vi "Open Document.vi"(7 "xwpfDocument Type":refnum<class "xwpfDocument.lvclass">, 8 "error in (no error)":errorcluster, 11 "Document Path":path) -> (0 "error out":errorcluster, 3 "xwpfDocument out":refnum<class "xwpfDocument.lvclass">)   [LabVIEW 2017, in "Word_Specific.lvlib" / "xwpfDocument.lvclass"]
uses:
  xwpfDocument.lvclass
  C:/Users/Neo/Desktop/Dev_Tools_BR/LabVIEW_NPOI/src/lib/NPOI 2.1.1/NPOI.OOXML.dll
  lib/NPOI 2.1.1/NPOI.OOXML.dll
  xwpfDocument.lvclass/xwpfDocument.ctl
  Support/File Stream/File Stream.lvlib
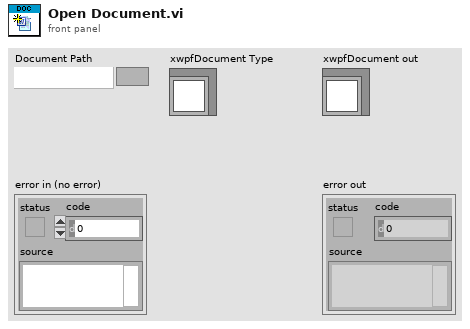
[diagram p1: front panel]
types:
  T1 = enum16{"Title", "Heading 1", "Heading 2", "Heading 3", "Normal", "Figure", "Page Break"}
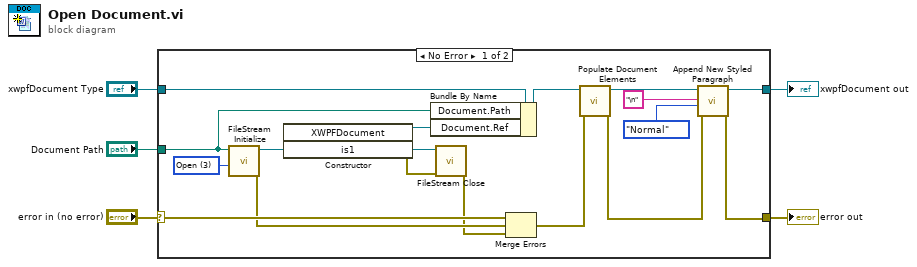
[diagram p0: block diagram]
diagram:
  n1 = case shown="No Error" "error in (no error)" {
    selector: "error in (no error)" -> [w21 w24]
    tunnel: [w8 w24] -> w4
    tunnel: [w10 w23] -> w2
    tunnel: "xwpfDocument Type" -> [w22 w23]
    tunnel: "Document Path" -> [w11 _]
    frame No Error {
      w20 = 3 items=["CreateNew"=1, "Create"=2, "Open"=3, "OpenOrCreate"=4, "Truncate"=5, "Append"=6] ("mode")
      n2 = call "FileStream Initialize.vi"("mode"=w20, "path"=w11) -> ("error out"=w16:errorcluster, "new reference"=w18:refnum<k24>)  [unwired: 8 in]
      n3 = constructor class="XWPFDocument"("is1"=w18) -> (reference out=w19:refnum<k24>, error out=w17:errorcluster)  [unwired: 3 in, 2 out]
      n4 = Bundle By Name(cluster=w22, "Document.Path"=w11, "Document.Ref"=w19) -> (w14:refnum<class "xwpfDocument.lvclass">)
      n5 = call "FileStream Close.vi"("error in (no error)"=w17, "reference"=w18) -> ("error out"=w15:errorcluster)  [unwired: 9 in]
      n6 = Merge Errors(w21, w16, w15) -> (w12:errorcluster)
      n7 = call "Populate Document Elements.vi"("error in (no error)"=w12, "xwpfDocument in"=w14) -> ("error out"=w9:errorcluster, "xwpfDocument out"=w13:refnum<class "xwpfDocument.lvclass">)  [unwired: 8 in]
      n8 = call "Append New Styled Paragraph.vi"("error in (no error)"=w9, "Type"=T1."Normal", "Paragraph.Text"="\n", "xwpfDocument in"=w13) -> ("error out"=w8:errorcluster, "xwpfDocument out"=w10:refnum<class "xwpfDocument.lvclass">)  [unwired: 6 in]
    }
    frame Error {
    }
  }
  "error out" <- w4
  "xwpfDocument out" <- w2
